vi "#62_MAV_MSG_NAV_CONTROLLER_OUTPUT_DECODE.vi"(11 "mavlink_payload":u8[](array[numeric])) -> (3 "NAV_CONTROLLER_OUTPUT":T1)   [LabVIEW 2023]
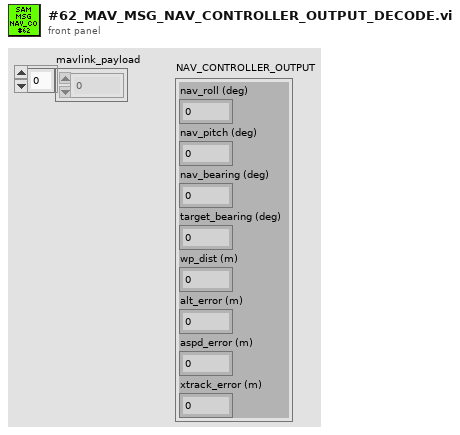
[diagram p1: front panel]
types:
  T1 = cluster{"nav_roll (deg)":sgl, "nav_pitch (deg)":sgl, "nav_bearing (deg)":i16, "target_bearing (deg)":i16, "wp_dist (m)":u16, "alt_error (m)":sgl, "aspd_error (m)":sgl, "xtrack_error (m)":sgl}
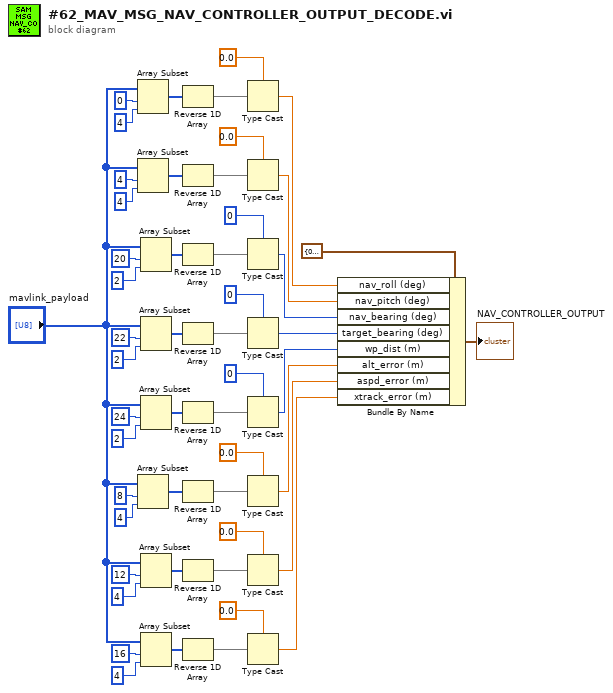
[diagram p0: block diagram]
diagram:
  n1 = Array Subset(array="mavlink_payload", index=0 ("Index"), length=4) -> (w50:u8[])
  n2 = Array Subset(array="mavlink_payload", index=4 ("Index"), length=4) -> (w42:u8[])
  n3 = Array Subset(array="mavlink_payload", index=8 ("Index"), length=4) -> (w18:u8[])
  n4 = Array Subset(array="mavlink_payload", index=20 ("Index"), length=2) -> (w36:u8[])
  n5 = Array Subset(array="mavlink_payload", index=22 ("Index"), length=2) -> (w30:u8[])
  n6 = Array Subset(array="mavlink_payload", index=24 ("Index"), length=2) -> (w24:u8[])
  n7 = Array Subset(array="mavlink_payload", index=12 ("Index"), length=4) -> (w12:u8[])
  n8 = Array Subset(array="mavlink_payload", index=16 ("Index"), length=4) -> (w6:u8[])
  n9 = Reverse 1D Array(array=w50) -> (reversed array=w49:u8[])
  n10 = Reverse 1D Array(array=w42) -> (reversed array=w41:u8[])
  n11 = Reverse 1D Array(array=w36) -> (reversed array=w35:u8[])
  n12 = Reverse 1D Array(array=w30) -> (reversed array=w29:u8[])
  n13 = Reverse 1D Array(array=w24) -> (reversed array=w23:u8[])
  n14 = Reverse 1D Array(array=w18) -> (reversed array=w17:u8[])
  n15 = Reverse 1D Array(array=w12) -> (reversed array=w11:u8[])
  n16 = Reverse 1D Array(array=w6) -> (reversed array=w5:u8[])
  n17 = Type Cast(type=sgl 0.0 ("Index"), x=w49) -> (*(type *) &x=w44:sgl)
  n18 = Type Cast(type=sgl 0.0 ("Index"), x=w41) -> (*(type *) &x=w38:sgl)
  n19 = Type Cast(type=i16 0 ("Index"), x=w35) -> (*(type *) &x=w32:i16)
  n20 = Type Cast(type=i16 0 ("Index"), x=w29) -> (*(type *) &x=w26:i16)
  n21 = Type Cast(type=u16 0 ("Index"), x=w23) -> (*(type *) &x=w20:u16)
  n22 = Type Cast(type=sgl 0.0 ("Index"), x=w17) -> (*(type *) &x=w14:sgl)
  n23 = Type Cast(type=sgl 0.0 ("Index"), x=w11) -> (*(type *) &x=w8:sgl)
  n24 = Type Cast(type=sgl 0.0 ("Index"), x=w5) -> (*(type *) &x=w1:sgl)
  n25 = Bundle By Name(cluster=T1 {"nav_roll (deg)"=0.0, "nav_pitch (deg)"=0.0, "nav_bearing (deg)"=0, "target_bearing (deg)"=0, "wp_dist (m)"=0, "alt_error (m)"=0.0, "aspd_error (m)"=0.0, "xtrack_error (m)"=0.0} ("NAV_CONTROLLER_OUTPUT"), "nav_roll (deg)"=w44, "nav_pitch (deg)"=w38, "nav_bearing (deg)"=w32, "target_bearing (deg)"=w26, "wp_dist (m)"=w20, "alt_error (m)"=w14, "aspd_error (m)"=w8, "xtrack_error (m)"=w1) -> (→"NAV_CONTROLLER_OUTPUT":T1)
